vi "Newest_CSV.vi"(8 "error in":errorcluster, 11 "Folder Path In":path) -> (0 "error out":errorcluster, 3 "File Path Out":path)   [LabVIEW 2019]
panel:
  # "Overview: This VI takes in a listing of files from a folder path, finds out all the files in the folder, and returns the path to the most recent file.\nRequirements: LabVIEW Base Development System\nInstructions:\n1. Select folder for searching most recent file.\n2. Run VI.\n3. Observe most recent file at File Path Out indicator."
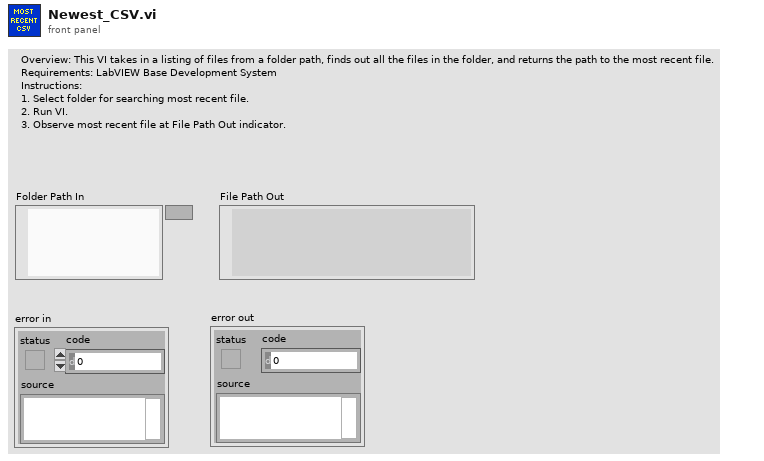
[diagram p1: front panel]
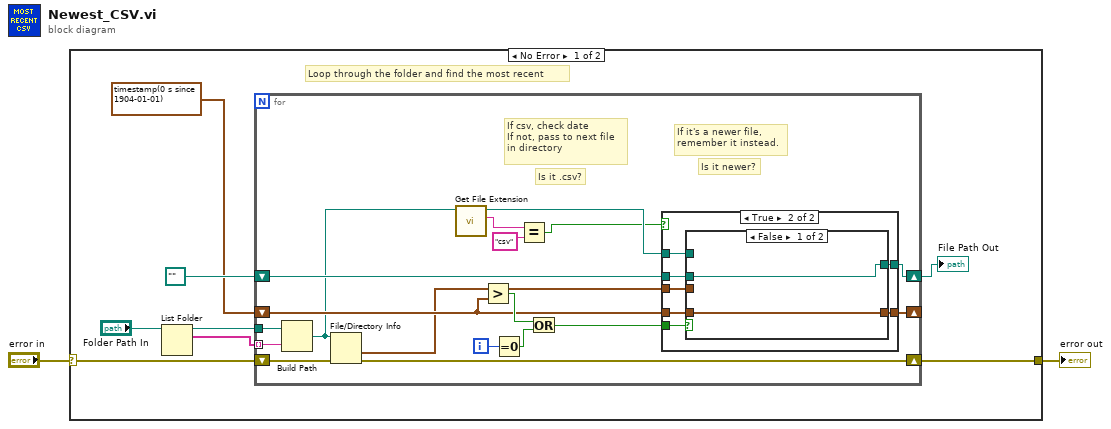
[diagram p0: block diagram]
diagram:
  n1 = case shown="No Error" "error in" {
    selector: "error in" -> [w6 w42]
    tunnel: [w10 w42] -> w2
    frame No Error {
      # "Loop through the folder and find the most recent"
      n2 = List Folder(path="Folder Path In") -> (path out=w3:path, filenames=w4:string[])  [unwired: 3 in, 2 out]
      n3 = for {
        shift-right: [w22] -> _
        shift-left: timestamp(0 s since 1904-01-01) ("last mod 2") -> [w23]
        shift-right: [w20] -> w9
        shift-left: path "" -> [w19]
        shift-right: [w18] -> w10
        shift-left: w6 -> [w28]
        tunnel: w4 -> [w17] mode=indexing
        tunnel: w3 -> [w16]
        i -> [w24]
        # "If csv, check date\nIf not, pass to next file \nin directory"
        # "Is it .csv?"
        # "Is it newer?"
        # "If it's a newer file,\nremember it instead."
        n4 = Build Path(base path=w16, name or relative path=w17) -> (appended path=w15:path)
        n5 = File/Directory Info(path=w15, error in=w28) -> (last mod=w21:timestamp, error out=w18:errorcluster)  [unwired: 5 out]
        n6 = call <vilib>:"Get File Extension.vi"("file"=w15) -> ("lowercase file extension"=w13:string, "dup file"=w14:path)  [unwired: 6 in, 3 out]
        n7 = Greater?(x=w21, y=w23) -> (0:w26:bool)
        n8 = Equal To 0?(x=w24) -> (x = 0?=w25:bool)
        n9 = Equal?(x=w13, y="csv") -> (x = y?=w11:bool)
        n10 = Or(x=w26, y=w25) -> (x .or. y?=w27:bool)
        n11 = case shown="True" w11 {
          tunnel: w27 -> [_ w37]
          tunnel: w23 -> [w29 w36]
          tunnel: [w29 w35] -> w22
          tunnel: w21 -> [_ w34]
          tunnel: [w30 w33] -> w20
          tunnel: w19 -> [w30 w32]
          tunnel: w14 -> [_ w31]
          frame False {
          }
          frame True {
            n12 = case shown="False" w37 {
              tunnel: w36 -> [w39 _]
              tunnel: [w39 w41] -> w35
              tunnel: w34 -> [_ w41]
              tunnel: w31 -> [_ w40]
              tunnel: [w38 w40] -> w33
              tunnel: w32 -> [w38 _]
              frame False {
              }
              frame True {
              }
            }
          }
        }
      }
      "File Path Out" <- w9
    }
    frame Error {
      # "If there is any error, do not do anything."
    }
  }
  "error out" <- w2
